vi "MotorEnable.vi"(8 "Error In":errorcluster, 10 "Enable?(F)":bool, 11 "Reference In":T1={"VISA resource name"="", "MotorType"=enum."AK80-64", "CAN ID"=1}) -> (0 "Error Out":errorcluster, 3 "Reference Out":T1={"VISA resource name"="", "MotorType"=enum."AK80-64", "CAN ID"=1})   [LabVIEW 2019, in "CubeMarsBLDClib.lvlib"]
uses:
  CubeMarsBLDClib.lvlib
  Reference.ctl
  MotorType.ctl
  MotorParameters.ctl
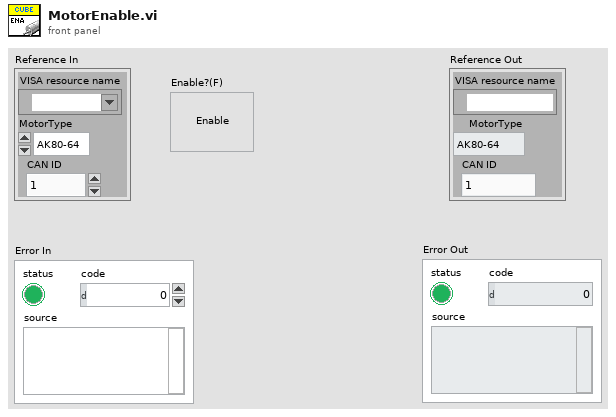
[diagram p1: front panel]
types:
  T1 = typedef "CubeMarsBLDClib.lvlib/Reference.ctl" = cluster{"VISA resource name":refnum<visa-resource-name>, "MotorType":T2, "CAN ID":u32}
  T2 = typedef "CubeMarsBLDClib.lvlib/MotorType.ctl" = enum16{"AK80-64", "AK80-9", "AK80-8", "AK80-6", "AK70-10", "AK60-6", "AK10-9"}
  T3 = typedef "CubeMarsBLDClib.lvlib/MotorParameters.ctl" = cluster{"Position(rad)":dbl, "Speed(rad/s)":dbl, "Kp":dbl, "Kd":dbl, "Torque (N.M)":dbl}
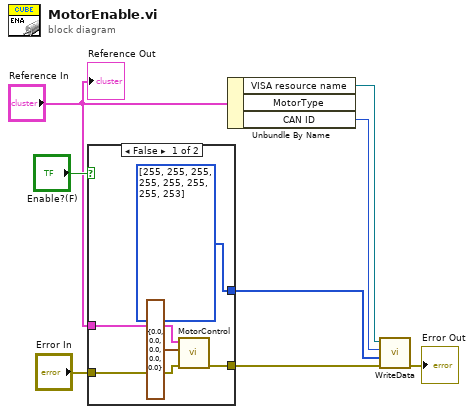
[diagram p0: block diagram]
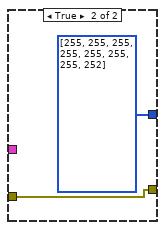
[diagram p2: hidden frame]
diagram:
  n1 = case shown="False" "Enable?(F)" {
    tunnel: [u8[] [255, 255, 255, 255, 255, 255, 255, 253] ("Data(0~8Byte) 2") u8[] [255, 255, 255, 255, 255, 255, 255, 252] ("Data(0~8Byte) 2")] -> w8
    tunnel: "Error In" -> [w11 w14]
    tunnel: [w10 w14] -> w2
    tunnel: "Reference In" -> [w9 _]
    frame False {
      n2 = call "MotorControl.vi"("error in"=w11, "ValueIn"=T3 {"Position(rad)"=0.0, "Speed(rad/s)"=0.0, "Kp"=0.0, "Kd"=0.0, "Torque (N.M)"=0.0}, "Reference In"=w9) -> ("error out"=w10:errorcluster)  [unwired: 6 in, 2 out]
    }
    frame True {
    }
  }
  n3 = Unbundle By Name("Reference In") -> ("VISA resource name"=w6:refnum<visa-resource-name>, "CAN ID"=w7:u32)  [unwired: 1 out]
  n4 = call "WriteData.vi"("error in"=w2, "Data(0~8Byte)"=w8, "ID"=w7, "VISA Refnum in"=w6) -> ("error out"=→"Error Out":errorcluster)  [unwired: 6 in, 1 out]
  "Reference Out" <- "Reference In"
